vi "Add User.vi"(0 "User Configuration Manager in":refnum<class "User Configuration Manager.lvclass">, 5 "Username":string, 11 "error in (no error)":errorcluster) -> (4 "User Configuration Manager out":refnum<class "User Configuration Manager.lvclass">, 8 "Replaced":bool, 15 "error out":errorcluster)   [LabVIEW 2017, in "User Configuration Manager.lvlib" / "User Configuration Manager.lvclass"]
uses:
  User Configuration Manager.lvclass
  User Configuration Manager.lvclass/User Configuration Manager.ctl
  cf98066f-11f4-4ec7-8ce1-afbc5e72ff21.vi
  Accessors/Read Linked List ID.vi
  Accessors/Read Linked List Ref .vi
  Read Encryption Type.vi
  <vilib>/gpm_packages/@cs/linked-list/Source/Linked List/ILinkedList/ILinked List.lvclass
  iEncryption/iEncryption.lvclass
  <vilib>/gpm_packages/@cs/linked-list/Source/Linked List/Linked List Ref/Linked List Ref.lvclass
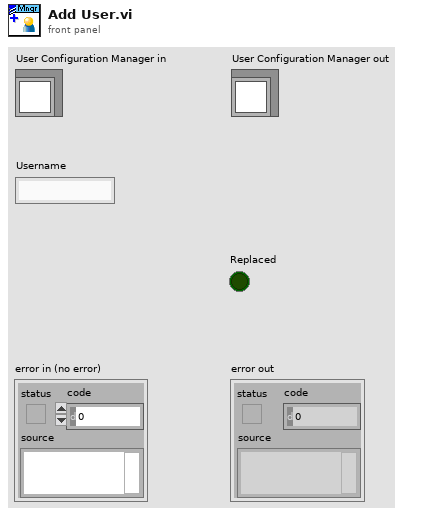
[diagram p1: front panel]
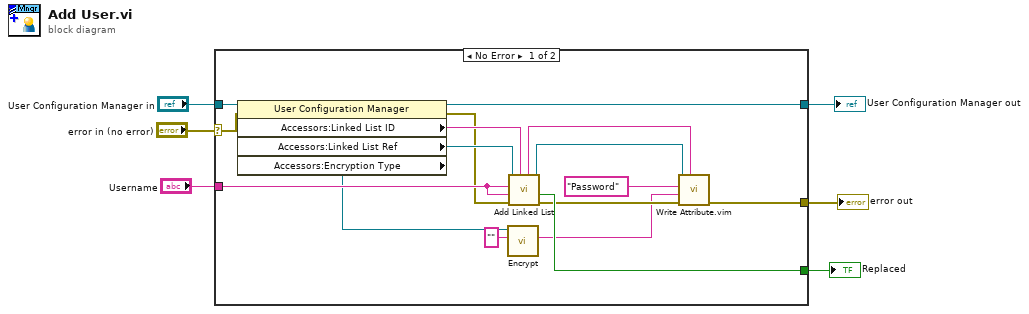
[diagram p0: block diagram]
diagram:
  n1 = case shown="No Error" "error in (no error)" {
    selector: "error in (no error)" -> [w20 w24]
    tunnel: "User Configuration Manager in" -> [w22 w23]
    tunnel: [w21 w23] -> w5
    tunnel: [w12 w24] -> w3
    tunnel: "Username" -> [w17 _]
    tunnel: [w16 _] -> w1
    frame No Error {
      n2 = property class="User Configuration Manager"(reference=w22, error in=w20) -> (reference out=w21:refnum<class "User Configuration Manager.lvclass">, error out=w15:errorcluster, "Accessors:Linked List ID"=w19:string, "Accessors:Linked List Ref "=w18:refnum<data-value>, "Accessors:Encryption Type"=w9:refnum<class "iEncryption.lvclass">)
      n3 = call-dynamic "Encrypt.vi"("String"="", "iEncryption in"=w9) -> ("Encrypted String"=w7:string)  [unwired: 9 in]
      n4 = call <vilib>:"Add Linked List.vi"("Parent ID"=w19, "error in (no error)"=w15, "Linked List ID"=w17, "Name"=w17, "Linked List Ref"=w18) -> ("error out"=w13:errorcluster, "Replaced?"=w16:bool, "Linked List Ref out"=w11:refnum<data-value>, "Linked List ID out"=w10:string)  [unwired: 3 in]
      n5 = call "Write Attribute.vim"("Linked List ID"=w10, "error in (no error)"=w13, "Attribute"=w7, "Attribute Name"="Password", "Linked List Ref"=w11) -> ("error out"=w12:errorcluster)  [unwired: 3 in, 3 out]
    }
    frame Error {
    }
  }
  "error out" <- w3
  "User Configuration Manager out" <- w5
  "Replaced" <- w1
